vi "multipart_upload.uninitialize_upload.vi"(11 "output cluster":T1) -> ()   [LabVIEW 2020, in "Nominal Client.lvclass"]
uses:
  Nominal Client.lvclass
  <vilib>/addons/_JKI.lib/REST Client/classes/REST Client/REST Client.lvclass
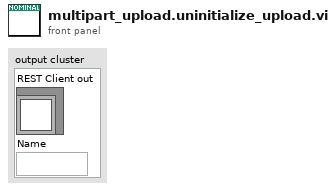
[diagram p1: front panel]
types:
  T1 = cluster{"REST Client out":refnum<class "REST Client.lvclass">, "Name":string}
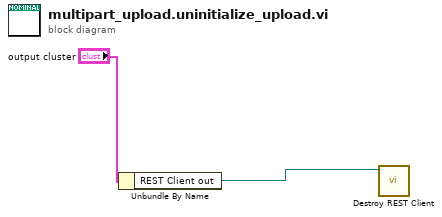
[diagram p0: block diagram]
diagram:
  n1 = Unbundle By Name("output cluster") -> ("REST Client out"=w1:refnum<class "REST Client.lvclass">)
  n2 = call-dynamic "Destroy REST Client.vi"("REST Client in"=w1) -> ()  [unwired: 10 in, 1 out]
